vi "O.vi"(11 "DataIn":T1) -> (3 "DataOut":T1)   [LabVIEW 2017]
doc: "SubVI criada para mostrar um popup para o usuário indicando que o player O é o ganhador.\n[Covers: REQ15]"
uses:
  controls/DataIn.ctl
  MatchDataClasses/MatchData/MatchData.lvclass
  controls/Tabuleiro.ctl
  controls/GameOption.ctl
  controls/Table.ctl
  Globals.vi
panel:
  in  "Sair":bool
  in  "Jogar Novamente":bool
  # "O é o vencedor!"
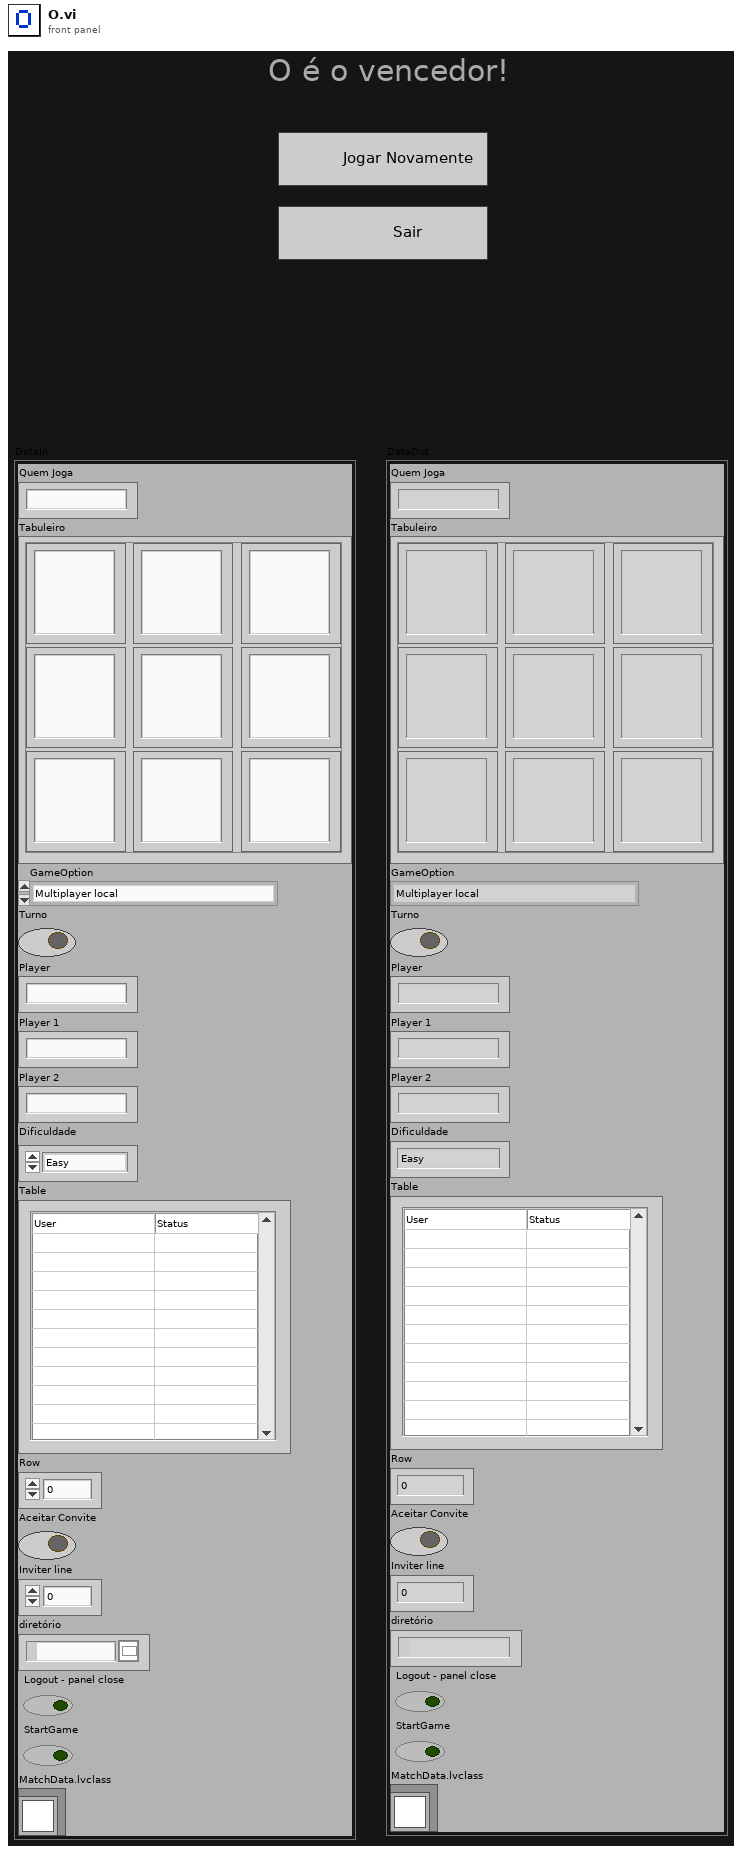
[diagram p1: front panel]
types:
  T1 = typedef "DataIn.ctl" = cluster{"Quem Joga":string, "Tabuleiro":T2, "GameOption":T3, "Turno":bool, "Player":string, "Player 1":string, "Player 2":string, "Dificuldade":enum16{"Easy", "Medium", "Hard"}, "Table":T4, "Row":u32, "Aceitar Convite":bool, "Inviter line":u32, "diretório":path, "Logout - panel close":bool, "StartGame":bool, "MatchData.lvclass":refnum<class "MatchData.lvclass">}
  T2 = typedef "Tabuleiro.ctl" = cluster{"(0,0)":string, "(1,0)":string, "(0,1)":string, "(1,1)":string, "(2,0)":string, "(1,2)":string, "(2,2)":string, "(0,2)":string, "(2,1) ":string}
  T3 = typedef "GameOption.ctl" = enum16{"Multiplayer local", "Multiplayer remoto", "Single Player", "Wait for Event", "Initialize", "Stop"}
  T4 = typedef "Table.ctl" = string[][]
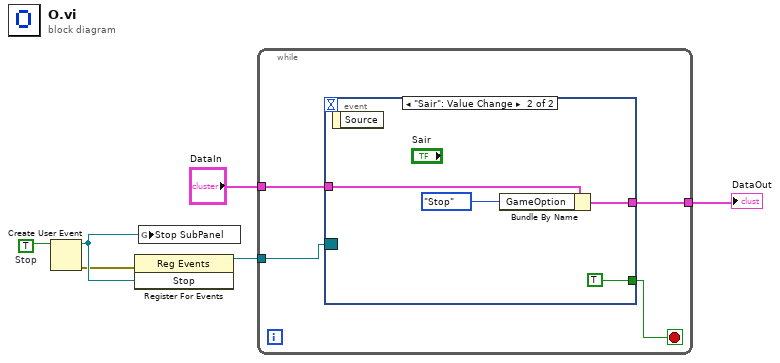
[diagram p0: block diagram]
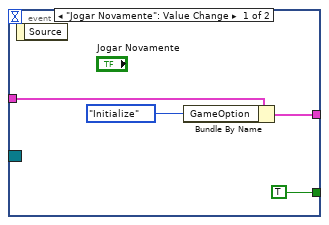
[diagram p2: hidden frame]
diagram:
  w3 = TRUE  # Stop
  n1 = Create User Event(user event datatype=w3) -> (user event=w4:refnum<user-event>, error out=w2:errorcluster)  [unwired: 1 in]
  n2 = register-events(error in=w2, w4) -> (reference out=w1:refnum<event-registration>)  [unwired: 1 in, 1 out]
  n3 = global write "Globals.vi" "Stop SubPanel"(w4) -> ()
  n4 = while {
    tunnel: "DataIn" -> [w9]
    tunnel: [w10] -> w5
    tunnel: w1 -> [w7]
    stop <- w8 stop-if-true
    n5 = event shown="[1] \"Sair\": Value Change" {
      selector: w7 -> [_ _]
      dyn-events: _ -> [_ _]
      timeout: _ -> [_ _]
      tunnel: [w12 w16] -> w10
      tunnel: w9 -> [w13 w17]
      tunnel: [TRUE TRUE] -> w8
      event "Jogar Novamente": Value Change {
        n6 = event-data() -> ()  [unwired: 1 in, 1 out]
        n7 = Bundle By Name(cluster=w13, "GameOption"=GameOption."Initialize") -> (w12:T1)
      }
      event "Sair": Value Change {
        n8 = event-data() -> ()  [unwired: 1 in, 1 out]
        n9 = Bundle By Name(cluster=w17, "GameOption"=GameOption."Stop") -> (w16:T1)
      }
    }
  }
  "DataOut" <- w5
